vi "Query Home Screen.vi"(8 "error IO":errorcluster, 11 "VISA resource name":refnum<visa-resource-name>) -> (0 "error Out":errorcluster, 2 "Home Screen":u16(ring) items=["Perform Tests", "Menu", "My Menu"], 3 "VISA resource Out":refnum<visa-resource-name>)   [LabVIEW 2016, in "eec EST 300.lvlib"]
doc: "SMM?\nReturns the Home Screen setting.\nHome Screen: Set the default screen upon instrument power up.\nThere are 3 options:\n0=Perform Tests\n1=Menu\n2=My Menu"
uses:
  <instrlib>/eec EST 300/eec EST 300.lvlib
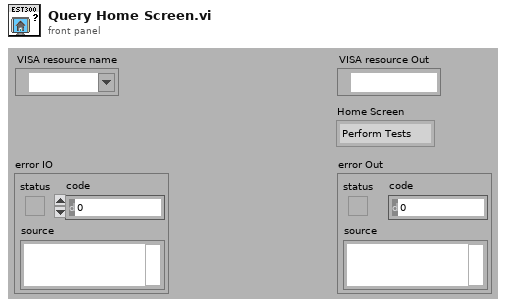
[diagram p1: front panel]
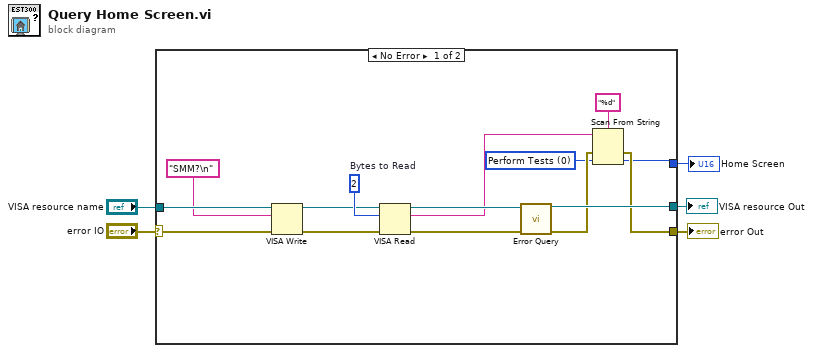
[diagram p0: block diagram]
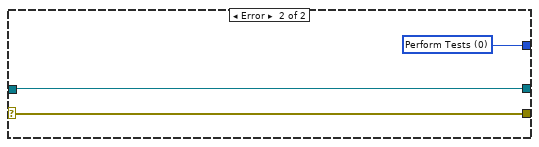
[diagram p2: hidden frame]
diagram:
  n1 = case shown="No Error" "error IO" {
    selector: "error IO" -> [w20 w23]
    tunnel: [w9 w23] -> w2
    tunnel: [w18 w22] -> w3
    tunnel: "VISA resource name" -> [w19 w22]
    tunnel: [w7 w21] -> w1
    frame No Error {
      w6 = u16 0 items=["Perform Tests", "Menu", "My Menu"] ("Home Screen")
      w14 = u32 2  # Bytes to Read
      n2 = VISA Write(VISA resource name=w19, write buffer="SMM?\n" ("Command to Send (empty)"), error in (no error)=w20) -> (VISA resource name out=w13:refnum<visa-resource-name>, error out=w12:errorcluster)  [unwired: 1 out]
      n3 = VISA Read(VISA resource name=w13, byte count=w14, error in (no error)=w12) -> (VISA resource name out=w16:refnum<visa-resource-name>, read buffer=w8:string, error out=w15:errorcluster)  [unwired: 1 out]
      n4 = call <instrlib>:"Error Query.vi"("VISA resource name"=w16, "error in (no error)"=w15) -> ("VISA resource name out"=w18:refnum<visa-resource-name>, "error out"=w10:errorcluster)  [unwired: 10 in, 2 out]
      n5 = Scan From String(format string="%d", input string=w8, error in=w10, default 1=w6) -> (error out=w9:errorcluster, output 1=w7:u16)  [unwired: 1 in, 2 out]
    }
    frame Error {
      w21 = u16 0 items=["Perform Tests", "Menu", "My Menu"] ("Home Screen")
    }
  }
  "VISA resource Out" <- w3
  "error Out" <- w2
  "Home Screen" <- w1
